vi "Add shared lock.vi"(8 "error in (no error)":errorcluster) -> (0 "error out":errorcluster)   [LabVIEW 2015, in "RefMem DMA Custom Device.lvlib"]
uses:
  RefMem DMA Custom Device.lvlib
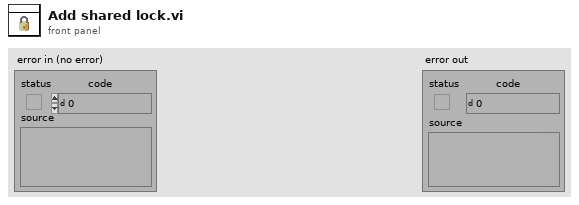
[diagram p1: front panel]
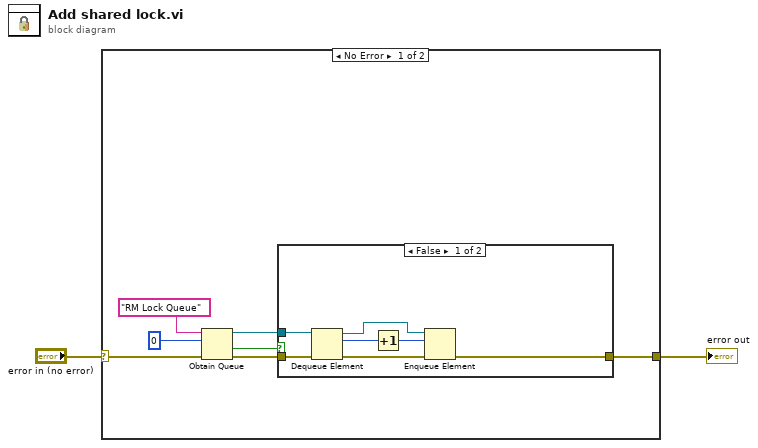
[diagram p0: block diagram]
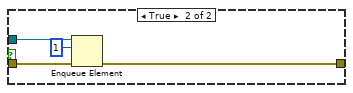
[diagram p2: hidden frame]
diagram:
  n1 = case shown="No Error" "error in (no error)" {
    selector: "error in (no error)" -> [w8 w21]
    tunnel: [w4 w21] -> w1
    frame No Error {
      n2 = Obtain Queue(name (unnamed)="RM Lock Queue", element data type=0, error in (no error)=w8) -> (queue out=w6:refnum<queue>, created new?=w7:bool, error out=w5:errorcluster)  [unwired: 2 in]
      n3 = case shown="False" w7 {
        tunnel: w6 -> [w16 w20]
        tunnel: w5 -> [w15 w18]
        tunnel: [w10 w17] -> w4
        frame False {
          n4 = Dequeue Element(queue=w16, error in (no error)=w15) -> (queue out=w13:refnum<queue>, element=w14:i32, error out=w12:errorcluster)  [unwired: 1 in, 1 out]
          n5 = Increment(x=w14) -> (x+1=w11:i32)
          n6 = Enqueue Element(queue=w13, element=w11, error in (no error)=w12) -> (error out=w10:errorcluster)  [unwired: 1 in, 2 out]
        }
        frame True {
          n7 = Enqueue Element(queue=w20, element=1, error in (no error)=w18) -> (error out=w17:errorcluster)  [unwired: 1 in, 2 out]
        }
      }
    }
    frame Error {
    }
  }
  "error out" <- w1
